vi "global_var.vi"() -> ()   [LabVIEW 2013]
panel:
  out "voltage measures":string
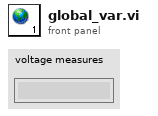
[diagram p1: front panel]
diagram:
